vi "BT数据判定.vi"(7 "data in":i16[](array[numeric])) -> (8 "result":bool)   [LabVIEW 2016]
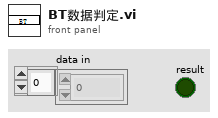
[diagram p1: front panel]
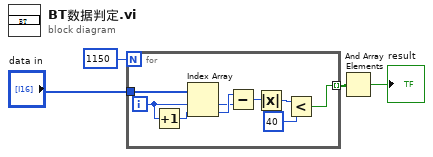
[diagram p0: block diagram]
diagram:
  n1 = for {
    N: 1150 -> [_]
    tunnel: "data in" -> [w13]
    tunnel: [w7] -> w3 mode=indexing
    i -> [w11]
    n2 = Increment(x=w11) -> (x+1=w12:i32)
    n3 = Index Array(array=w13, index #1=w11, index #2=w12) -> (element #1=w9:i16, element #2=w10:i16)
    n4 = Subtract(x=w10, y=w9) -> (x-y=w6:i16)
    n5 = Absolute Value(x=w6) -> (abs(x)=w5:i16)
    n6 = Less?(x=w5, y=u16 40) -> (x < y?=w7:bool)
  }
  n7 = And Array Elements(Boolean array=w3) -> (logical AND=→"result":bool)
